vi "CreatePrivateEvents.vi"(8 "error in (no error)":errorcluster, 11 "DAQmx(AI)":refnum<class "DAQmx(AI).lvclass">) -> (0 "error out":errorcluster, 3 "DAQmx(AI) out":refnum<class "DAQmx(AI).lvclass">)   [LabVIEW 2019, in "DAQmx(AI).lvclass"]
doc: "JKI State Machine Objects (SMO) 1.1.8.32\nJKI - JKI\nCopyright (c) 2016, JKI"
uses:
  DAQmx(AI).lvclass
  Typedefs/Logging--Cluster.ctl
  DAQmx(AI).lvclass/DAQmx(AI).ctl
  vi.lib/JKI/JKI SMO/SMO/SMO.lvclass
panel:
  # "For instructions on how to use the JKI State Machine Objects, examples and video tutorials, visit:\nhttp://jki.net/state-machine-objects/\n\nJKI State Machine Objects™\nhttp://jki.net/state-machine-objects/\nCopyright (C) 2005-2015, JKI <info@jki.net>\nALL RIGHTS RESERVED"
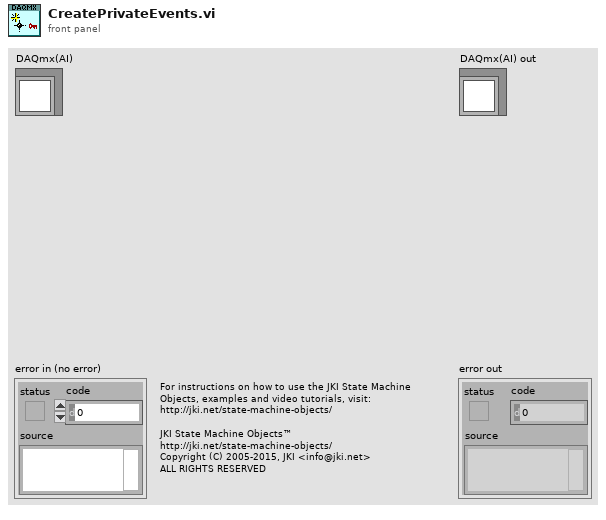
[diagram p1: front panel]
types:
  T1 = typedef "DAQmx(AI).lvclass/Logging--Cluster.ctl" = cluster{"TDMS File Path":path, "Group Name":string}
  T2 = typedef "DAQmx(AI).lvclass/PrivateData--Ref.ctl" = refnum<data-value>
  T3 = typedef "DAQmx(AI).lvclass/PrivateData--Cluster.ctl" = cluster{"Configuration":T4, "Public Events":T6, "Data":dbl, "Scaling":T7, "Private Events":T13}
  T4 = typedef "DAQmx(AI).lvclass/Configuration--Cluster.ctl" = cluster{"PhysChan":tag, "Period (ms)":i64, "input terminal cfg":i32, "minimum value":dbl, "maximum value":dbl, "units":T5, "task name":string, "TDMS File Path":path, "Group Name":string}
  T5 = typedef "DAQmx(AI).lvclass/Units -- Enum.ctl" = enum16{"Volts", "Amps", "Deg F", "Deg C", "Deg R", "Kelvins", "Strain", "Ohms", "Hz", "Seconds", "Meters", "Inches", "Degrees", "Radians", "Ticks", "g", "m/s^2", "m/s", "in/s", "Pascals", "Newtons", "Pounds", "kgf", "psi", "bar", "Nm", "oz-in", "lb-in", "lb-ft", "Volts/Volt", "mVolts/Volt", "From TEDS"}
  T6 = typedef "DAQmx(AI).lvclass/PublicEvents--Cluster.ctl" = cluster{"Value Changed":refnum<user-event>, "Task Configuration":refnum<user-event>, "Scaling":refnum<user-event>}
  T7 = typedef "DAQmx(AI).lvclass/Scaling--Cluster.ctl" = cluster{"Scale Name":string, "Scale Type":T8, "Scaled Units":string, "Linear":T9, "Map Range":T10, "Polynomial":T11, "Table":T12}
  T8 = typedef "DAQmx(AI).lvclass/ScalingType--Enum.ctl" = enum16{"No scaling", "Linear", "Map Range", "Polynomial", "Table"}
  T9 = typedef "DAQmx(AI).lvclass/Scaling(Linear)--Cluster.ctl" = cluster{"Slope":dbl, "Intercept":dbl}
  T10 = typedef "DAQmx(AI).lvclass/Scaling(MapRange)--Cluster.ctl" = cluster{"Minimum":dbl, "Maximum":dbl}
  T11 = typedef "DAQmx(AI).lvclass/Scaling(Polynomial)--Cluster.ctl" = cluster{"forward coeff":dbl[], "reverse coeff":dbl[]}
  T12 = typedef "DAQmx(AI).lvclass/Scaling(Table)--Cluster.ctl" = cluster{"scaled values":dbl[], "pres-scaled values":dbl[]}
  T13 = typedef "DAQmx(AI).lvclass/PrivateEvents--Cluster.ctl" = cluster{"Logging":refnum<user-event>}
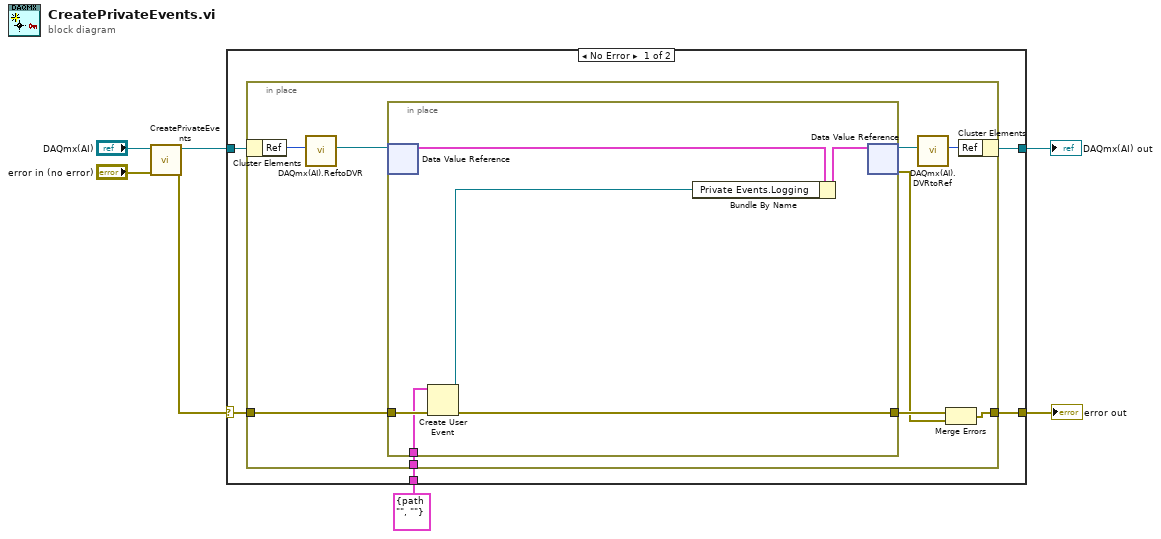
[diagram p0: block diagram]
diagram:
  n1 = call-parent "CreatePrivateEvents.vi"("error in (no error)"="error in (no error)", "SMO"="DAQmx(AI)") -> ("error out"=w4:errorcluster, "SMO out"=w5:refnum<class "DAQmx(AI).lvclass">)  [unwired: 8 in]
  n2 = case shown="No Error" w4 {
    selector: w4 -> [w10 w29]
    tunnel: [w9 w29] -> w1
    tunnel: [w11 w28] -> w2
    tunnel: w5 -> [w12 w28]
    tunnel: T1 {"TDMS File Path"=path "", "Group Name"=""} ("Logging") -> [w8 _]
    frame No Error {
      n3 = in-place {
        in-place-border: w10 -> [w21]
        in-place-border: [w18] -> w9
        in-place-border: w8 -> [w17]
        n4 = in-place-cluster #1(w12) -> ("Ref"=w16:u32)
        n5 = call "DAQmx(AI).ReftoDVR.vi"("Ref"=w16) -> ("Ref"=w15:T2)  [unwired: 10 in]
        n6 = in-place {
          in-place-border: w21 -> [w25]
          in-place-border: [w22] -> w20
          in-place-border: w17 -> [w24]
          n7 = in-place-dvr #2(w15) -> (w26:T3)  [unwired: 1 out]
          n8 = Create User Event(user event datatype=w24, error in=w25) -> (user event=w23:refnum<user-event>, error out=w22:errorcluster)
          n9 = Bundle By Name(cluster=w26, "Private Events.Logging"=w23) -> (w27:T3)
          n10 = in-place-dvr #2(w27) -> (w14:T2, w19:errorcluster)
        }
        n11 = call "DAQmx(AI).DVRtoRef.vi"("Ref"=w14) -> ("Ref"=w13:u32)  [unwired: 10 in]
        n12 = Merge Errors(w20, w19) -> (w18:errorcluster)
        n13 = in-place-cluster #1("Ref"=w13) -> (w11:refnum<class "DAQmx(AI).lvclass">)
      }
    }
    frame Error {
    }
  }
  "error out" <- w1
  "DAQmx(AI) out" <- w2
